vi "FixJKIHelper.vi"() -> ()   [LabVIEW 2014]
uses:
  <vilib>/Utility/miscctls.llb/LVRowAndColumnUnsignedTypeDef.ctl
panel:
  out "Multicolumn Listbox":i32(listbox)
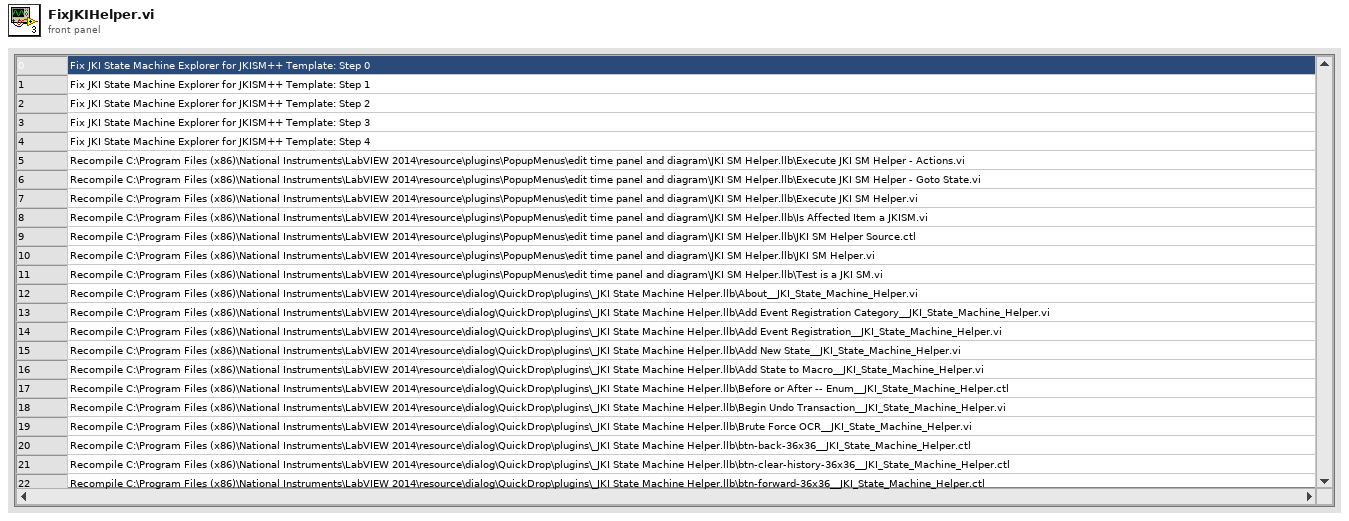
[diagram p1: front panel]
types:
  T1 = typedef "LVRowAndColumnUnsignedTypeDef.ctl" = cluster{"Row":u32, "Column":u32}
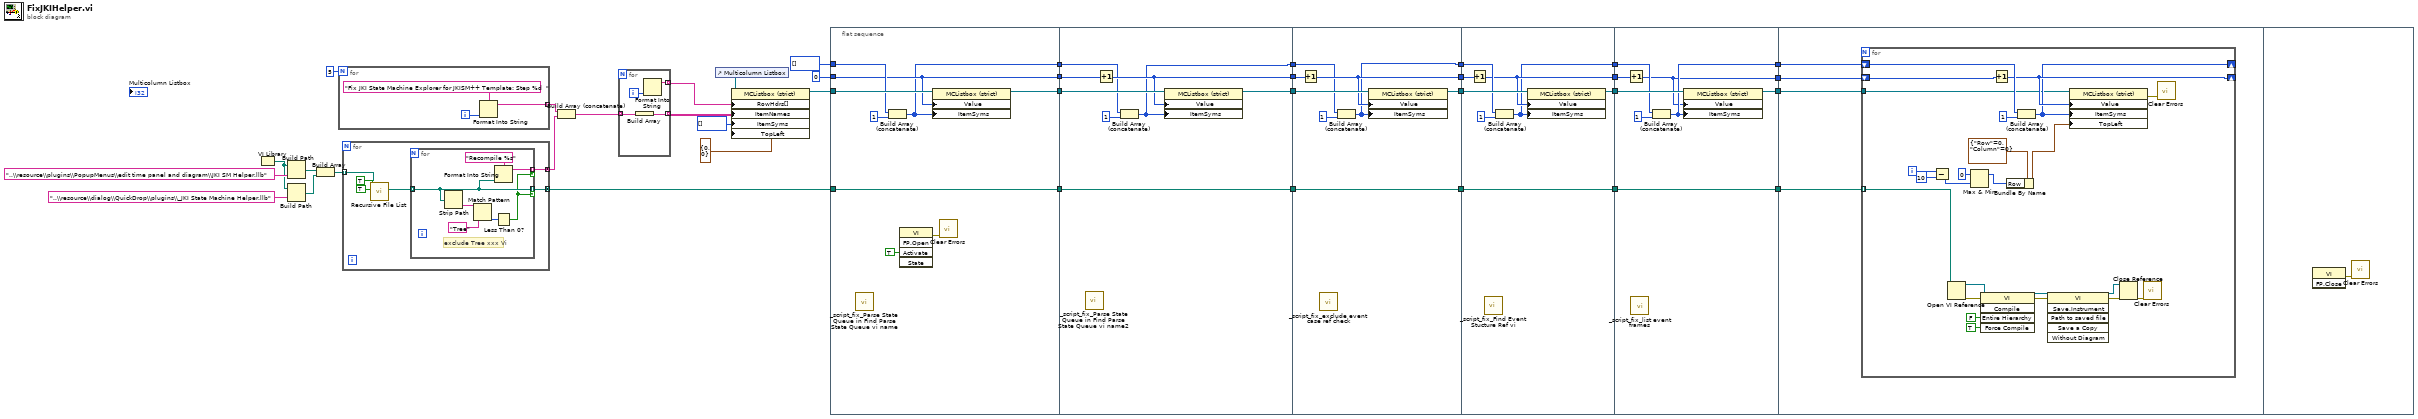
[diagram p0: block diagram]
diagram:
  n1 = VI Library() -> (path=w38:path)
  n2 = Build Path(base path=w38, name or relative path="..\\resource\\plugins\\PopupMenus\\edit time panel and diagram\\JKI SM Helper.llb") -> (appended path=w36:path)
  n3 = Build Path(base path=w38, name or relative path="..\\resource\\dialog\\QuickDrop\\plugins\\_JKI State Machine Helper.llb") -> (appended path=w34:path)
  n4 = Build Array(w36, w34) -> (w35:path[])
  n5 = for {
    N: 5 -> [_]
    tunnel: [w40] -> w26 mode=indexing
    i -> [w41]
    n6 = Format Into String(format string="Fix JKI State Machine Explorer for JKISM++ Template: Step %d  ", w41) -> (resulting string=w40:string)  [unwired: 2 in, 1 out]
  }
  n7 = for {
    tunnel: w35 -> [w46] mode=indexing
    tunnel: [w44] -> w28 mode=concatenating
    tunnel: [w43] -> w25 mode=concatenating
    n8 = call <vilib>:"Recursive File List.vi"("Continue Recursing on Error? (F)"=TRUE, "Treat LLBs as Folders?"=TRUE, "Folder Path"=w46) -> ("All Files in Dir"=w45:path[])  [unwired: 4 in, 4 out]
    n9 = for {
      tunnel: w45 -> [w51] mode=indexing
      tunnel: [w51] -> w44 mode=indexing if=w49
      tunnel: [w50] -> w43 mode=indexing if=w49
      # "exclude Tree xxx Vi"
      n10 = Strip Path(path=w51) -> (name=w55:string)  [unwired: 1 out]
      n11 = Match Pattern(string=w55, regular expression="Tree") -> (offset past match=w53:i32)  [unwired: 1 in, 3 out]
      n12 = Format Into String(format string="Recompile %s", w51) -> (resulting string=w50:string)  [unwired: 2 in, 1 out]
      n13 = Less Than 0?(x=w53) -> (x < 0?=w49:bool)
    }
  }
  n14 = Build Array (concatenate)(w26, w25) -> (w24:string[])
  n15 = for {
    tunnel: w24 -> [w57] mode=indexing
    tunnel: [w58] -> w22 mode=indexing
    tunnel: [w56] -> w21 mode=indexing
    i -> [w59]
    n16 = Build Array(w57) -> (w56:string[])
    n17 = Format Into String(w59) -> (resulting string=w58:string)  [unwired: 3 in, 1 out]
  }
  n18 = control-ref of="Multicolumn Listbox"() -> (w23:refnum<vi>)
  n19 = property class="MCListbox (strict)"(reference=w23, "RowHdrs[]"=w22, "ItemNames"=w21, "ItemSyms"=i32[] [] ("Item Symbols"), "TopLeft"=T1 {"Row"=0, "Column"=0} ("Top Left Visible Cell")) -> (reference out=w20:refnum<vi>)  [unwired: 1 in, 1 out]
  n20 = flat-sequence {
    tunnel: [w68] -> w29
    tunnel: w28 -> [w68]
    tunnel: w20 -> [w67]
    tunnel: 0 -> [w63]
    tunnel: i32[] [] ("Item Symbols") -> [w65]
    tunnel: [w64] -> w16
    tunnel: [w63] -> w15
    tunnel: [w62] -> w14
    tunnel: [w76] -> w30
    tunnel: w29 -> [w76]
    tunnel: w16 -> [w74]
    tunnel: w15 -> [w73]
    tunnel: w14 -> [w70]
    tunnel: [w72] -> w13
    tunnel: [w71] -> w12
    tunnel: [w69] -> w11
    tunnel: [w84] -> w31
    tunnel: w30 -> [w84]
    tunnel: w13 -> [w82]
    tunnel: w12 -> [w81]
    tunnel: w11 -> [w78]
    tunnel: [w80] -> w10
    tunnel: [w79] -> w9
    tunnel: [w77] -> w8
    tunnel: [w92] -> w32
    tunnel: w31 -> [w92]
    tunnel: w10 -> [w90]
    tunnel: w9 -> [w89]
    tunnel: w8 -> [w88]
    tunnel: [w87] -> w7
    tunnel: [w86] -> w6
    tunnel: [w85] -> w5
    tunnel: [w100] -> w33
    tunnel: w32 -> [w100]
    tunnel: w7 -> [w98]
    tunnel: w6 -> [w97]
    tunnel: w5 -> [w96]
    tunnel: [w95] -> w4
    tunnel: [w94] -> w3
    tunnel: [w93] -> w2
    tunnel: w33 -> [w104]
    tunnel: w4 -> [w103]
    tunnel: w3 -> [w102]
    tunnel: w2 -> [w101]
    frame #0 {
      n21 = call "_script_fix_Parse State Queue in Find Parse State Queue vi name.vi"() -> ()  [unwired: 12 in]
      n22 = Build Array (concatenate)(w65, 1) -> (w62:i32[])
      n23 = invoke class="VI" method="FP.Open"("Activate"=TRUE ("Activate?")) -> (error out=w61:errorcluster)  [unwired: 4 in, 4 out]
      n24 = property class="MCListbox (strict)"(reference=w67, "Value"=w63, "ItemSyms"=w62) -> (reference out=w64:refnum<vi>)  [unwired: 1 in, 1 out]
      n25 = call <vilib>:"Clear Errors.vi"("error in (no error)"=w61) -> ()  [unwired: 6 in, 1 out]
    }
    frame #1 {
      n26 = call "_script_fix_Parse State Queue in Find Parse State Queue vi name2.vi"() -> ()  [unwired: 12 in]
      n27 = Increment(x=w73) -> (x+1=w71:i32)
      n28 = Build Array (concatenate)(w70, 1) -> (w69:i32[])
      n29 = property class="MCListbox (strict)"(reference=w74, "Value"=w71, "ItemSyms"=w69) -> (reference out=w72:refnum<vi>)  [unwired: 1 in, 1 out]
    }
    frame #2 {
      n30 = Increment(x=w81) -> (x+1=w79:i32)
      n31 = call "_script_fix_exclude event case ref check.vi"() -> ()  [unwired: 12 in]
      n32 = Build Array (concatenate)(w78, 1) -> (w77:i32[])
      n33 = property class="MCListbox (strict)"(reference=w82, "Value"=w79, "ItemSyms"=w77) -> (reference out=w80:refnum<vi>)  [unwired: 1 in, 1 out]
    }
    frame #3 {
      n34 = Increment(x=w89) -> (x+1=w87:i32)
      n35 = call "_script_fix_Find Event Stucture Ref vi.vi"() -> ()  [unwired: 12 in]
      n36 = Build Array (concatenate)(w88, 1) -> (w85:i32[])
      n37 = property class="MCListbox (strict)"(reference=w90, "Value"=w87, "ItemSyms"=w85) -> (reference out=w86:refnum<vi>)  [unwired: 1 in, 1 out]
    }
    frame #4 {
      n38 = Increment(x=w98) -> (x+1=w94:i32)
      n39 = call "_script_fix_list event frames.vi"() -> ()  [unwired: 12 in]
      n40 = Build Array (concatenate)(w96, 1) -> (w95:i32[])
      n41 = property class="MCListbox (strict)"(reference=w97, "Value"=w94, "ItemSyms"=w95) -> (reference out=w93:refnum<vi>)  [unwired: 1 in, 1 out]
    }
    frame #5 {
      n42 = for {
        tunnel: w104 -> [w128] mode=indexing
        shift-right: [w115] -> _
        shift-left: w102 -> [w116]
        shift-right: [w114] -> _
        shift-left: w103 -> [w117]
        tunnel: w101 -> [w113]
        i -> [w109]
        n43 = Subtract(x=w109, y=10) -> (x-y=w110:i32)
        n44 = Open VI Reference(vi path=w128) -> (vi reference=w124:refnum<vi>, error out=w125:errorcluster)  [unwired: 5 in]
        n45 = Max & Min(x=0, y=w110) -> (max(x,y)=w106:i32)  [unwired: 1 out]
        n46 = invoke class="VI" method="Compile"(reference=w124, error in=w125, "Entire Hierarchy"=FALSE ("Compile Entire Hierarchy (F)"), "Force Compile"=TRUE ("Force Compile (T)")) -> (reference out=w123:refnum<vi>, error out=w122:errorcluster)  [unwired: 1 in, 3 out]
        n47 = Increment(x=w116) -> (x+1=w115:i32)
        n48 = Bundle By Name(cluster=T1 {"Row"=0, "Column"=0} ("Top Left Visible Cell"), "Row"=w106) -> (w111:T1)
        n49 = Build Array (concatenate)(w117, 1) -> (w114:i32[])
        n50 = invoke class="VI" method="Save.Instrument"(reference=w123, error in=w122) -> (reference out=w120:refnum<vi>, error out=w121:errorcluster)  [unwired: 4 in, 4 out]
        n51 = property class="MCListbox (strict)"(reference=w113, "Value"=w115, "ItemSyms"=w114, "TopLeft"=w111) -> (error out=w105:errorcluster)  [unwired: 1 in, 1 out]
        n52 = Close Reference(reference=w120, error in (no error)=w121) -> (error out=w119:errorcluster)
        n53 = call <vilib>:"Clear Errors.vi"("error in (no error)"=w119) -> ()  [unwired: 6 in, 1 out]
        n54 = call <vilib>:"Clear Errors.vi"("error in (no error)"=w105) -> ()  [unwired: 6 in, 1 out]
      }
    }
    frame #6 {
      n55 = invoke class="VI" method="FP.Close"() -> (error out=w129:errorcluster)  [unwired: 3 in, 2 out]
      n56 = call <vilib>:"Clear Errors.vi"("error in (no error)"=w129) -> ()  [unwired: 6 in, 1 out]
    }
  }
